vi "Begin.vi"(8 "error in":errorcluster) -> (0 "error out":errorcluster)   [LabVIEW 2020]
doc: "Called before other user functions, this VI is expected to open initial I/O refnums, load in file data, and do all program initialization. Notice that the <B>error out</B> terminal is simply used for data flow. Wiring it to other structures or subVIs ensures that this VI runs first."
uses:
  <vilib>/Rock Robotics/WPI/DriverStation/WPI_DriverStationRobotMode2.ctl
  <vilib>/Rock Robotics/WPI/Joystick/WPI_JoystickDeviceEnum.ctl
  <vilib>/Rock Robotics/WPI/ThirdParty/Phoenix-LabVIEW/Motor Controller/Controls/CTRE_Phoenix_MotorControl_ControlMode.ctl
  <vilib>/Rock Robotics/SystemInterfaces/AI/FPGA_AIChannel.ctl
  Robot Global Data.vi
  <vilib>/Rock Robotics/Network Tables/NT Write String Array.vi
panel:
  in  "Boolean":bool
  out "Voltage BL":dbl
  out "Voltage BR":dbl
  out "Voltage FL":dbl
  out "Voltage FR":dbl
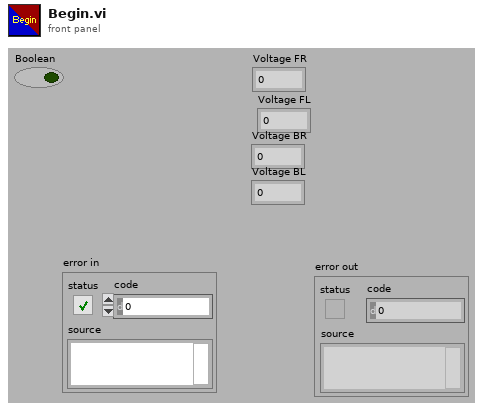
[diagram p1: front panel]
types:
  T1 = typedef "FPGA_AIChannel.ctl" = enum8{"AI 0", "AI 1", "AI 2", "AI 3", "AI MXP 0", "AI MXP 1", "AI MXP 2", "AI MXP 3", "Invalid"}
  T2 = typedef "CTRE_Phoenix_MotorControl_ControlMode.ctl" = u16
  T3 = typedef "WPI_JoystickDeviceEnum.ctl" = enum16{"USB 0", "USB 1", "USB 2", "USB 3", "USB 4", "USB 5"}
  T4 = typedef "WPI_DriverStationRobotMode2.ctl" = enum16{"Autonomous Disabled", "Autonomous Enabled", "Teleop Disabled", "Teleop Enabled", "Disconnected", "Finish", "Test Disabled", "Test Enabled", "Emergency Stopped"}
  T5 = typedef "WPI_AnalogChannelDevRef.ctl" = cluster{"DevStatus":errorcluster, "Analog Channel":T1}
  T6 = typedef "WPI_MotorControlDeviceRef.ctl" = cluster{"DeviceStatus":errorcluster, "Type":T7, "PWM":cluster{"PWM Channel":T8, "DeadBand":T9}, "CAN":cluster{"Device Number":u8, "SetOutput VI Ref":variant, "GetOutput VI Ref":variant, "Enable VI Ref":variant, "Disable VI Ref":variant, "Data":variant}, "Invert":bool, "DIO PWM":cluster{"PWM \"Enable\" Channel":T8, "DIOChannel":T10, "PWM Rate":dbl}}
  T7 = typedef "WPI_MotorControlType.ctl" = enum16{"PWM", "CAN", "DIO PWM"}
  T8 = typedef "FPGA_DIOPWMChannel.ctl" = enum8{"PWM 0", "PWM 1", "PWM 2", "PWM 3", "PWM 4", "PWM 5", "PWM 6", "PWM 7", "PWM 8", "PWM 9", "PWM MXP 0", "PWM MXP 1", "PWM MXP 2", "PWM MXP 3", "PWM MXP 4", "PWM MXP 5", "PWM MXP 6", "PWM MXP 7", "PWM MXP 8", "PWM MXP 9", "Invalid"}
  T9 = typedef "WPI_PWMDeadband.ctl" = cluster{"Name":string, "maxPositivePwm":i32, "minPositivePwm":i32, "centerPwm":i32, "maxNegativePwm":i32, "minNegativePwm":i32, "angularRange":u16}
  T10 = typedef "FPGA_DIOChannel.ctl" = enum8{"DIO 0", "DIO 1", "DIO 2", "DIO 3", "DIO 4", "DIO 5", "DIO 6", "DIO 7", "DIO 8", "DIO 9", "DIO MXP 0", "DIO MXP 1", "DIO MXP 2", "DIO MXP 3", "DIO MXP 4", "DIO MXP 5", "DIO MXP 6", "DIO MXP 7", "DIO MXP 8", "DIO MXP 9", "DIO MXP 10", "DIO MXP 11", "DIO MXP 12", "DIO MXP 13", "DIO MXP 14", "DIO MXP 15", "SPI Port CS1", "SPI Port CS2", "SPI Port CS3", "SPI Port MISO", "SPI Port MOSI", "Invalid"}
  T11 = typedef "WPI_JoystickDevRef.ctl" = cluster{"Device":T3}
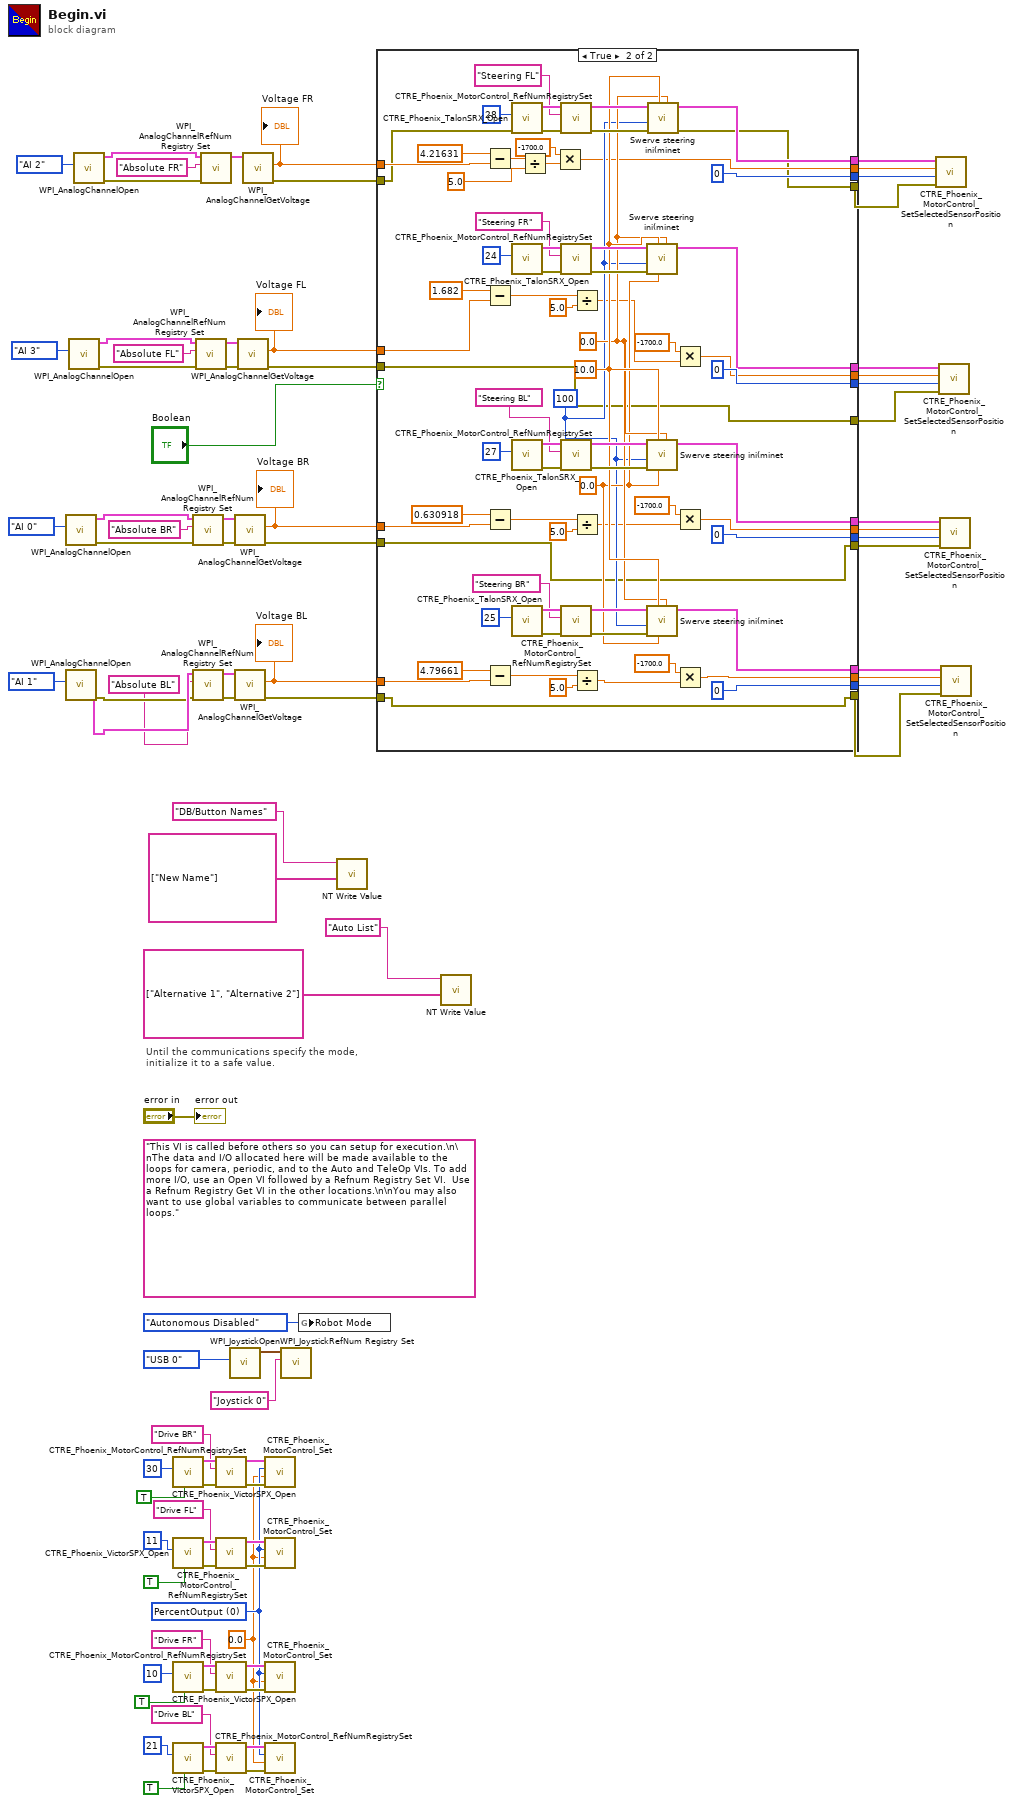
[diagram p0: block diagram]
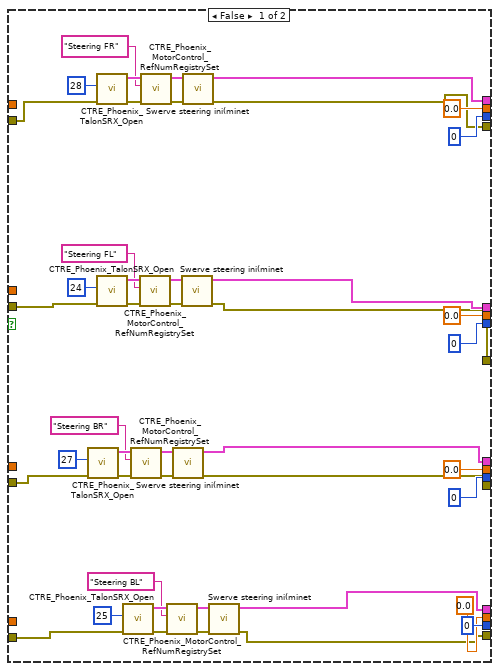
[diagram p2: hidden frame]
diagram:
  w53 = 0.0 ("Output")
  w54 = T2 0 items=["PercentOutput"=0, "Position"=1, "Velocity"=2, "Current"=3, "Follower"=5, "MotionProfile"=6, "MotionMagic"=7, "MotionProfileArc"=10, "Disabled"=15] ("Control Mode")
  (unwired) "This VI is called before others so you can setup for execution.\n\nThe data and I/O allocated here will be made available to the loops for camera, periodic, and to the Auto and TeleOp VIs. To add more I/O, use an Open VI followed by a Refnum Registry Set VI.  Use a Refnum Registry Get VI in the other locations.\n\nYou may also want to use global variables to communicate between parallel loops."
  # "Until the communications specify the mode,\ninitialize it to a safe value."
  n1 = call <vilib>:"WPI_AnalogChannelOpen.vi"("Analog Channel"=FPGA_AIChannel."AI 0") -> ("error out"=w36:errorcluster, "AIDeviceRef"=w37:T5)  [unwired: 9 in]
  n2 = call <vilib>:"WPI_AnalogChannelOpen.vi"("Analog Channel"=FPGA_AIChannel."AI 1") -> ("error out"=w40:errorcluster, "AIDeviceRef"=w41:T5)  [unwired: 9 in]
  n3 = call <vilib>:"WPI_AnalogChannelOpen.vi"("Analog Channel"=FPGA_AIChannel."AI 3") -> ("error out"=w44:errorcluster, "AIDeviceRef"=w45:T5)  [unwired: 9 in]
  n4 = call <vilib>:"WPI_AnalogChannelOpen.vi"("Analog Channel"=FPGA_AIChannel."AI 2") -> ("error out"=w48:errorcluster, "AIDeviceRef"=w49:T5)  [unwired: 9 in]
  n5 = call <vilib>:"CTRE_Phoenix_VictorSPX_Open.vi"("Invert"=TRUE, "Device Number"=u8 30) -> ("error out"=w70:errorcluster, "PhoenixMotorControlDevRef"=w72:T6)  [unwired: 8 in]
  n6 = call <vilib>:"CTRE_Phoenix_VictorSPX_Open.vi"("Invert"=TRUE, "Device Number"=u8 11) -> ("error out"=w64:errorcluster, "PhoenixMotorControlDevRef"=w66:T6)  [unwired: 8 in]
  n7 = call <vilib>:"CTRE_Phoenix_VictorSPX_Open.vi"("Invert"=TRUE, "Device Number"=u8 10) -> ("error out"=w58:errorcluster, "PhoenixMotorControlDevRef"=w60:T6)  [unwired: 8 in]
  n8 = call <vilib>:"CTRE_Phoenix_VictorSPX_Open.vi"("Invert"=TRUE, "Device Number"=u8 21) -> ("error out"=w76:errorcluster, "PhoenixMotorControlDevRef"=w78:T6)  [unwired: 8 in]
  n9 = call <vilib>:"WPI_AnalogChannelRefNum Registry Set.vi"("error in (no error)"=w36, "refnum name"="Absolute BR", "AIDeviceRef"=w37) -> ("error out"=w33:errorcluster, "AIDeviceRef"=w34:T5)  [unwired: 7 in]
  n10 = call <vilib>:"WPI_AnalogChannelRefNum Registry Set.vi"("error in (no error)"=w40, "refnum name"="Absolute BL", "AIDeviceRef"=w41) -> ("error out"=w29:errorcluster, "AIDeviceRef"=w30:T5)  [unwired: 7 in]
  n11 = call <vilib>:"WPI_AnalogChannelRefNum Registry Set.vi"("error in (no error)"=w44, "refnum name"="Absolute FL", "AIDeviceRef"=w45) -> ("error out"=w27:errorcluster, "AIDeviceRef"=w28:T5)  [unwired: 7 in]
  n12 = call <vilib>:"WPI_AnalogChannelRefNum Registry Set.vi"("error in (no error)"=w48, "refnum name"="Absolute FR", "AIDeviceRef"=w49) -> ("AIDeviceRef"=w26:T5)  [unwired: 7 in, 1 out]
  n13 = call <vilib>:"CTRE_Phoenix_MotorControl_RefNumRegistrySet.vi"("error in (no error)"=w70, "refnum name"="Drive BR", "PhoenixMotorControlDevRef"=w72) -> ("error out"=w67:errorcluster, "PhoenixMotorControlDevRef"=w68:T6)  [unwired: 7 in]
  n14 = call <vilib>:"CTRE_Phoenix_MotorControl_RefNumRegistrySet.vi"("error in (no error)"=w64, "refnum name"="Drive FL", "PhoenixMotorControlDevRef"=w66) -> ("error out"=w61:errorcluster, "PhoenixMotorControlDevRef"=w62:T6)  [unwired: 7 in]
  n15 = call <vilib>:"CTRE_Phoenix_MotorControl_RefNumRegistrySet.vi"("error in (no error)"=w58, "refnum name"="Drive FR", "PhoenixMotorControlDevRef"=w60) -> ("error out"=w55:errorcluster, "PhoenixMotorControlDevRef"=w56:T6)  [unwired: 7 in]
  n16 = call <vilib>:"CTRE_Phoenix_MotorControl_RefNumRegistrySet.vi"("error in (no error)"=w76, "refnum name"="Drive BL", "PhoenixMotorControlDevRef"=w78) -> ("error out"=w73:errorcluster, "PhoenixMotorControlDevRef"=w74:T6)  [unwired: 7 in]
  n17 = call <vilib>:"WPI_JoystickOpen.vi"("JoystickDevice"=WPI_JoystickDeviceEnum."USB 0") -> ("JoystickDevRef"=w85:T11)  [unwired: 10 in]
  n18 = call <vilib>:"WPI_AnalogChannelGetVoltage.vi"("error in (no error)"=w33, "AIDeviceRef"=w34) -> ("error out"=w6:errorcluster, "Voltage"=w32:dbl)  [unwired: 7 in, 1 out]
  "Voltage BR" <- w32
  n19 = call <vilib>:"WPI_AnalogChannelGetVoltage.vi"("error in (no error)"=w29, "AIDeviceRef"=w30) -> ("error out"=w4:errorcluster, "Voltage"=w17:dbl)  [unwired: 7 in, 1 out]
  "Voltage BL" <- w17
  n20 = call <vilib>:"WPI_AnalogChannelGetVoltage.vi"("error in (no error)"=w27, "AIDeviceRef"=w28) -> ("error out"=w8:errorcluster, "Voltage"=w20:dbl)  [unwired: 7 in, 1 out]
  "Voltage FL" <- w20
  n21 = call <vilib>:"WPI_AnalogChannelGetVoltage.vi"("AIDeviceRef"=w26) -> ("error out"=w10:errorcluster, "Voltage"=w23:dbl)  [unwired: 8 in, 1 out]
  "Voltage FR" <- w23
  n22 = call <vilib>:"CTRE_Phoenix_MotorControl_Set.vi"("error in (no error)"=w67, "Output"=w53, "Control Mode"=w54, "PhoenixMotorControlDevRef"=w68) -> ()  [unwired: 6 in, 2 out]
  n23 = call <vilib>:"CTRE_Phoenix_MotorControl_Set.vi"("error in (no error)"=w61, "Output"=w53, "Control Mode"=w54, "PhoenixMotorControlDevRef"=w62) -> ()  [unwired: 6 in, 2 out]
  n24 = call <vilib>:"CTRE_Phoenix_MotorControl_Set.vi"("error in (no error)"=w55, "Output"=w53, "Control Mode"=w54, "PhoenixMotorControlDevRef"=w56) -> ()  [unwired: 6 in, 2 out]
  n25 = call <vilib>:"CTRE_Phoenix_MotorControl_Set.vi"("error in (no error)"=w73, "Output"=w53, "Control Mode"=w54, "PhoenixMotorControlDevRef"=w74) -> ()  [unwired: 6 in, 2 out]
  n26 = call <vilib>:"WPI_JoystickRefNum Registry Set.vi"("refnum name"="Joystick 0", "JoystickDevRef"=w85) -> ()  [unwired: 8 in, 2 out]
  n27 = global write "Robot Global Data.vi" "Robot Mode"(WPI_DriverStationRobotMode2."Autonomous Disabled" ("Robot Mode")) -> ()
  n28 = call-poly <vilib>:"NT Write Value.vi"("String Array"=string[] ["New Name"], "Name"="DB/Button Names") -> ()  [unwired: 9 in, 1 out]
  n29 = case shown="True" "Boolean" {
    tunnel: w32 -> [_ w172]
    tunnel: [w89 w171] -> w31
    tunnel: [u32 0 ("pidLoopIdx") u32 0 ("pidLoopIdx")] -> w25
    tunnel: [0.0 w164] -> w24
    tunnel: w23 -> [_ w163]
    tunnel: [u32 0 ("pidLoopIdx") u32 0 ("pidLoopIdx")] -> w22
    tunnel: [0.0 w156] -> w21
    tunnel: w20 -> [_ w155]
    tunnel: [u32 0 ("pidLoopIdx") u32 0 ("pidLoopIdx")] -> w19
    tunnel: [0.0 w149] -> w18
    tunnel: w17 -> [_ w147]
    tunnel: [u32 0 ("pidLoopIdx") u32 0 ("pidLoopIdx")] -> w16
    tunnel: [0.0 w140] -> w15
    tunnel: [w102 w139] -> w14
    tunnel: [w99 w138] -> w13
    tunnel: [w93 w137] -> w12
    tunnel: w10 -> [w127 w135]
    tunnel: [w95 w136] -> w9
    tunnel: w8 -> [w122 w134]
    tunnel: [w97 w134] -> w7
    tunnel: w6 -> [w113 w133]
    tunnel: [w90 w133] -> w5
    tunnel: w4 -> [w108 w132]
    tunnel: [w88 w132] -> w3
    frame False {
      n30 = call <vilib>:"CTRE_Phoenix_TalonSRX_Open.vi"("error in"=w113, "Device Number"=u8 27) -> ("error out"=w116:errorcluster, "PhoenixMotorControlDevRef"=w117:T6)  [unwired: 8 in]
      n31 = call <vilib>:"CTRE_Phoenix_TalonSRX_Open.vi"("error in"=w127, "Device Number"=u8 28) -> ("error out"=w130:errorcluster, "PhoenixMotorControlDevRef"=w131:T6)  [unwired: 8 in]
      n32 = call <vilib>:"CTRE_Phoenix_TalonSRX_Open.vi"("error in"=w122, "Device Number"=u8 24) -> ("error out"=w125:errorcluster, "PhoenixMotorControlDevRef"=w126:T6)  [unwired: 8 in]
      n33 = call <vilib>:"CTRE_Phoenix_TalonSRX_Open.vi"("error in"=w108, "Device Number"=u8 25) -> ("error out"=w111:errorcluster, "PhoenixMotorControlDevRef"=w112:T6)  [unwired: 8 in]
      n34 = call <vilib>:"CTRE_Phoenix_MotorControl_RefNumRegistrySet.vi"("error in (no error)"=w116, "refnum name"="Steering BR", "PhoenixMotorControlDevRef"=w117) -> ("error out"=w91:errorcluster, "PhoenixMotorControlDevRef"=w92:T6)  [unwired: 7 in]
      n35 = call <vilib>:"CTRE_Phoenix_MotorControl_RefNumRegistrySet.vi"("error in (no error)"=w125, "refnum name"="Steering FL", "PhoenixMotorControlDevRef"=w126) -> ("error out"=w98:errorcluster, "PhoenixMotorControlDevRef"=w100:T6)  [unwired: 7 in]
      n36 = call <vilib>:"CTRE_Phoenix_MotorControl_RefNumRegistrySet.vi"("error in (no error)"=w130, "refnum name"="Steering FR", "PhoenixMotorControlDevRef"=w131) -> ("error out"=w96:errorcluster, "PhoenixMotorControlDevRef"=w94:T6)  [unwired: 7 in]
      n37 = call <vilib>:"CTRE_Phoenix_MotorControl_RefNumRegistrySet.vi"("error in (no error)"=w111, "refnum name"="Steering BL", "PhoenixMotorControlDevRef"=w112) -> ("error out"=w101:errorcluster, "PhoenixMotorControlDevRef"=w103:T6)  [unwired: 7 in]
      n38 = call "Swerve steering ini(minet.vi"("error in (no error)"=w91, "PhoenixMotorControlDevRef In"=w92) -> ("error out"=w90:errorcluster, "PhoenixMotorControlDevRef Out"=w89:T6)  [unwired: 8 in]
      n39 = call "Swerve steering ini(minet.vi"("error in (no error)"=w98, "PhoenixMotorControlDevRef In"=w100) -> ("error out"=w97:errorcluster, "PhoenixMotorControlDevRef Out"=w99:T6)  [unwired: 8 in]
      n40 = call "Swerve steering ini(minet.vi"("error in (no error)"=w96, "PhoenixMotorControlDevRef In"=w94) -> ("error out"=w95:errorcluster, "PhoenixMotorControlDevRef Out"=w93:T6)  [unwired: 8 in]
      n41 = call "Swerve steering ini(minet.vi"("error in (no error)"=w101, "PhoenixMotorControlDevRef In"=w103) -> ("error out"=w88:errorcluster, "PhoenixMotorControlDevRef Out"=w102:T6)  [unwired: 8 in]
    }
    frame True {
      w174 = 0.0 ("D")
      w175 = 0.0 ("I")
      w176 = 10.0 ("P")
      w173 = u32 100 ("timeoutMs")
      n42 = Subtract(x=4.21631 ("Voltage"), y=w163) -> (x-y=w168:dbl)
      n43 = Subtract(x=1.682 ("Voltage"), y=w155) -> (x-y=w160:dbl)
      n44 = Subtract(x=0.630918 ("Voltage"), y=w172) -> (x-y=w144:dbl)
      n45 = Subtract(x=4.79661 ("Voltage"), y=w147) -> (x-y=w153:dbl)
      n46 = call <vilib>:"CTRE_Phoenix_TalonSRX_Open.vi"("error in"=w135, "Device Number"=u8 28) -> ("error out"=w199:errorcluster, "PhoenixMotorControlDevRef"=w200:T6)  [unwired: 8 in]
      n47 = call <vilib>:"CTRE_Phoenix_TalonSRX_Open.vi"("Device Number"=u8 24) -> ("error out"=w187:errorcluster, "PhoenixMotorControlDevRef"=w188:T6)  [unwired: 9 in]
      n48 = call <vilib>:"CTRE_Phoenix_TalonSRX_Open.vi"("Device Number"=u8 27) -> ("error out"=w191:errorcluster, "PhoenixMotorControlDevRef"=w192:T6)  [unwired: 9 in]
      n49 = call <vilib>:"CTRE_Phoenix_TalonSRX_Open.vi"("Device Number"=u8 25) -> ("error out"=w195:errorcluster, "PhoenixMotorControlDevRef"=w196:T6)  [unwired: 9 in]
      n50 = Divide(x=w168, y=5.0) -> (x/y=w167:dbl)
      n51 = Multiply(x=-1700.0, y=w167) -> (x*y=w164:dbl)
      n52 = call <vilib>:"CTRE_Phoenix_MotorControl_RefNumRegistrySet.vi"("error in (no error)"=w199, "refnum name"="Steering FL", "PhoenixMotorControlDevRef"=w200) -> ("error out"=w183:errorcluster, "PhoenixMotorControlDevRef"=w184:T6)  [unwired: 7 in]
      n53 = call <vilib>:"CTRE_Phoenix_MotorControl_RefNumRegistrySet.vi"("error in (no error)"=w187, "refnum name"="Steering FR", "PhoenixMotorControlDevRef"=w188) -> ("error out"=w181:errorcluster, "PhoenixMotorControlDevRef"=w182:T6)  [unwired: 7 in]
      n54 = call <vilib>:"CTRE_Phoenix_MotorControl_RefNumRegistrySet.vi"("error in (no error)"=w191, "refnum name"="Steering BL", "PhoenixMotorControlDevRef"=w192) -> ("error out"=w179:errorcluster, "PhoenixMotorControlDevRef"=w180:T6)  [unwired: 7 in]
      n55 = call <vilib>:"CTRE_Phoenix_MotorControl_RefNumRegistrySet.vi"("error in (no error)"=w195, "refnum name"="Steering BR", "PhoenixMotorControlDevRef"=w196) -> ("error out"=w177:errorcluster, "PhoenixMotorControlDevRef"=w178:T6)  [unwired: 7 in]
      n56 = Divide(x=w160, y=5.0) -> (x/y=w159:dbl)
      n57 = Divide(x=w144, y=5.0) -> (x/y=w143:dbl)
      n58 = Divide(x=w153, y=5.0) -> (x/y=w152:dbl)
      n59 = call "Swerve steering ini(minet.vi"("I"=w175, "D"=w174, "P"=w176, "error in (no error)"=w181, "timeoutMs"=w173, "PhoenixMotorControlDevRef In"=w182) -> ("PhoenixMotorControlDevRef Out"=w138:T6)  [unwired: 4 in, 1 out]
      n60 = call "Swerve steering ini(minet.vi"("I"=w175, "D"=w174, "P"=w176, "error in (no error)"=w179, "timeoutMs"=w173, "PhoenixMotorControlDevRef In"=w180) -> ("PhoenixMotorControlDevRef Out"=w171:T6)  [unwired: 4 in, 1 out]
      n61 = call "Swerve steering ini(minet.vi"("I"=w175, "D"=w174, "P"=w176, "error in (no error)"=w177, "timeoutMs"=w173, "PhoenixMotorControlDevRef In"=w178) -> ("PhoenixMotorControlDevRef Out"=w139:T6)  [unwired: 4 in, 1 out]
      n62 = call "Swerve steering ini(minet.vi"("I"=w175, "P"=w176, "error in (no error)"=w183, "timeoutMs"=w173, "PhoenixMotorControlDevRef In"=w184) -> ("error out"=w136:errorcluster, "PhoenixMotorControlDevRef Out"=w137:T6)  [unwired: 5 in]
      n63 = Multiply(x=-1700.0, y=w159) -> (x*y=w156:dbl)
      n64 = Multiply(x=-1700.0, y=w143) -> (x*y=w140:dbl)
      n65 = Multiply(x=-1700.0, y=w152) -> (x*y=w149:dbl)
    }
  }
  n66 = call-poly <vilib>:"NT Write Value.vi"("String Array"=string[] ["Alternative 1", "Alternative 2"], "Name"="Auto List") -> ()  [unwired: 9 in, 1 out]
  n67 = call <vilib>:"CTRE_Phoenix_MotorControl_SetSelectedSensorPosition.vi"("error in (no error)"=w9, "pidLoopIdx"=w25, "New Sensor Position"=w24, "PhoenixMotorControlDevRef"=w12) -> ()  [unwired: 6 in, 2 out]
  n68 = call <vilib>:"CTRE_Phoenix_MotorControl_SetSelectedSensorPosition.vi"("error in (no error)"=w7, "pidLoopIdx"=w22, "New Sensor Position"=w21, "PhoenixMotorControlDevRef"=w13) -> ()  [unwired: 6 in, 2 out]
  n69 = call <vilib>:"CTRE_Phoenix_MotorControl_SetSelectedSensorPosition.vi"("error in (no error)"=w5, "pidLoopIdx"=w16, "New Sensor Position"=w15, "PhoenixMotorControlDevRef"=w31) -> ()  [unwired: 6 in, 2 out]
  n70 = call <vilib>:"CTRE_Phoenix_MotorControl_SetSelectedSensorPosition.vi"("error in (no error)"=w3, "pidLoopIdx"=w19, "New Sensor Position"=w18, "PhoenixMotorControlDevRef"=w14) -> ()  [unwired: 6 in, 2 out]
  "error out" <- "error in"
